vi "ini_object_save.vi"(7 "generate error if unsuppoted data type (true)":bool=TRUE, 8 "error in":errorcluster, 10 "auto ini row":T1, 11 "refnum in":T2) -> (0 "error out":errorcluster, 3 "refnum out":T2)   [LabVIEW 2020]
uses:
  <vilib>/Utility/config.llb/Config Data RefNum.ctl
  ini_parse_row.ctl
  <vilib>/Utility/config.llb/Write Key (String).vi
  <vilib>/Utility/config.llb/Write Key (Path).vi
  <vilib>/Utility/config.llb/Write Key (Boolean).vi
  <vilib>/Utility/config.llb/Write Key (I32).vi
  <vilib>/Utility/config.llb/Write Key (Double).vi
  <vilib>/Utility/config.llb/Write Key (U32).vi
  <vilib>/Utility/config.llb/NI_LVConfig.lvlib
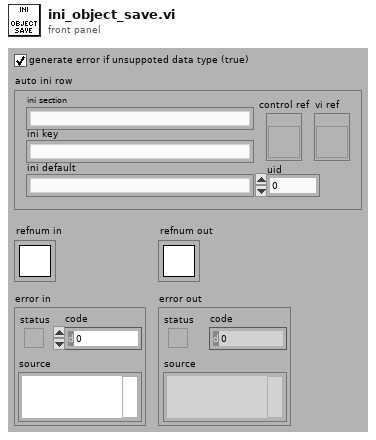
[diagram p1: front panel]
types:
  T1 = typedef "ini_parse_row.ctl" = cluster{"ini section":string, "ini key":string, "ini default":string, "control ref":refnum<vi>, "uid":i32, "vi ref":refnum<vi>}
  T2 = typedef "NI_LVConfig.lvlib/Config Data RefNum.ctl" = refnum<k1>
  T3 = cluster{"Value":string[][], "Row Headers[]":string[], "Column Headers[]":string[]}
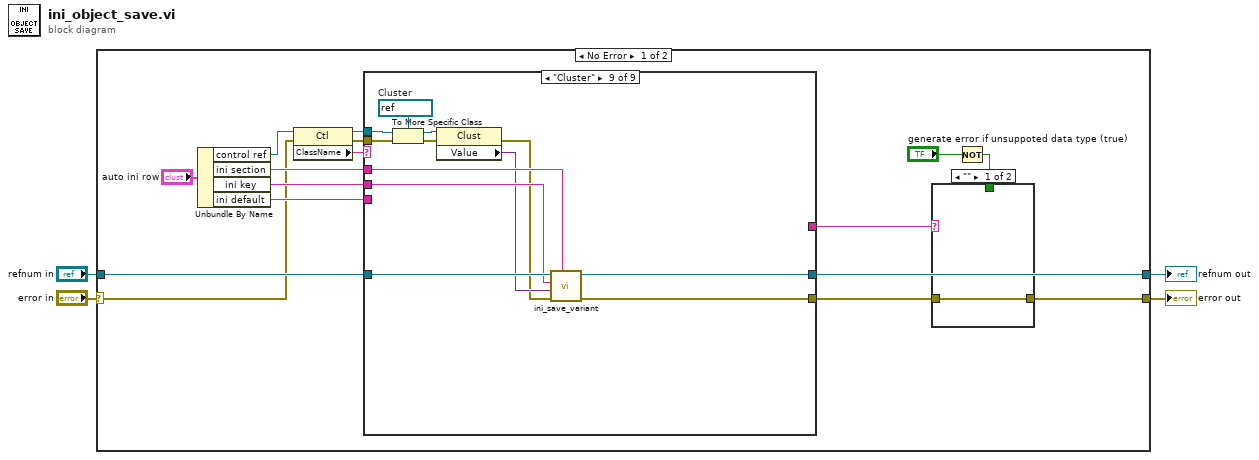
[diagram p0: block diagram]
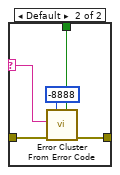
[diagram p2: hidden frame]
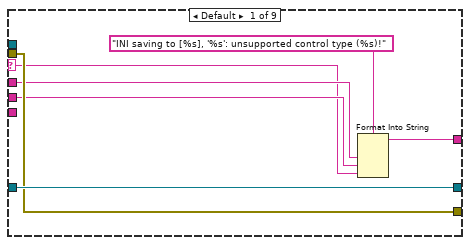
[diagram p3: hidden frame]
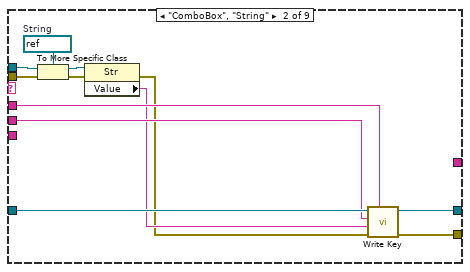
[diagram p4: hidden frame]
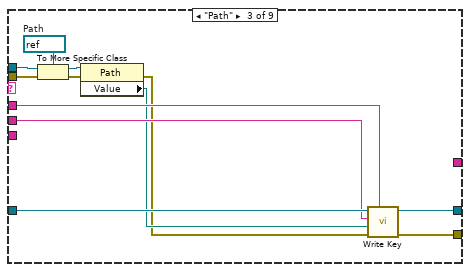
[diagram p5: hidden frame]
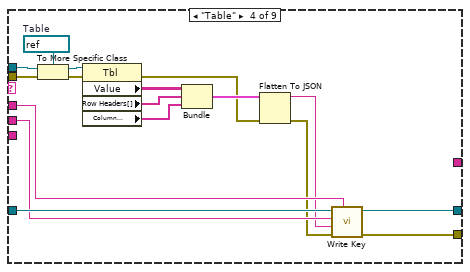
[diagram p6: hidden frame]
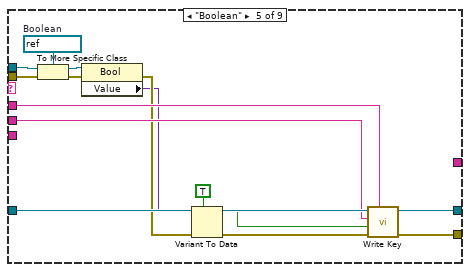
[diagram p7: hidden frame]
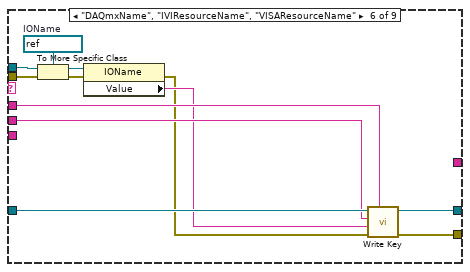
[diagram p8: hidden frame]
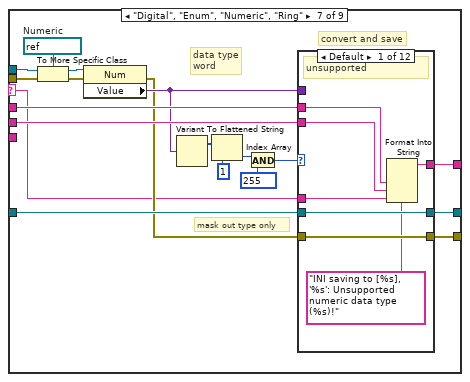
[diagram p9: hidden frame]
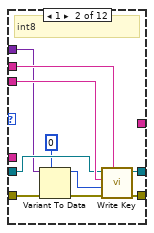
[diagram p10: hidden frame]
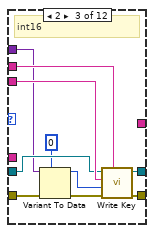
[diagram p11: hidden frame]
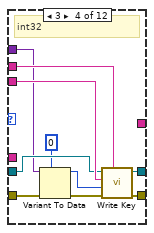
[diagram p12: hidden frame]
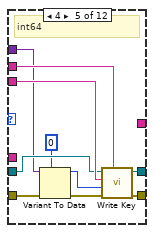
[diagram p13: hidden frame]
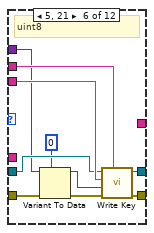
[diagram p14: hidden frame]
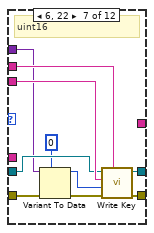
[diagram p15: hidden frame]
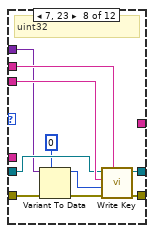
[diagram p16: hidden frame]
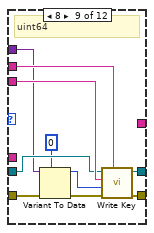
[diagram p17: hidden frame]
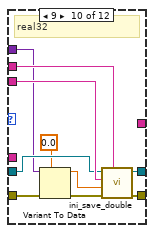
[diagram p18: hidden frame]
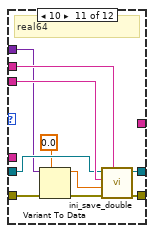
[diagram p19: hidden frame]
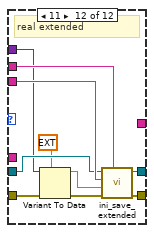
[diagram p20: hidden frame]
diagram:
  n1 = case shown="No Error" "error in" {
    selector: "error in" -> [w5 w424]
    tunnel: "refnum in" -> [w20 w423]
    tunnel: [w19 w423] -> w3
    tunnel: [w9 w424] -> w2
    frame No Error {
      n2 = Unbundle By Name("auto ini row") -> ("control ref"=w15:refnum<vi>, "ini section"=w17:string, "ini key"=w16:string, "ini default"=w13:string)
      n3 = property class="Ctl"(reference=w15, error in=w5) -> (reference out=w11:refnum<vi>, error out=w12:errorcluster, "ClassName"=w14:string)
      n4 = case shown="\"Cluster\"" w14 {
        selector: w14 -> [w27 _ _ _ _ _ w102 w243 _]
        tunnel: [w32 w45 w57 w74 w89 w101 w120 w253 w422] -> w10
        tunnel: w20 -> [w33 w44 w56 w73 w88 w100 w119 w252 w421]
        tunnel: [w33 w43 w55 w72 w87 w99 w118 w251 w420] -> w19
        tunnel: w17 -> [w29 w42 w54 w71 w86 w98 w117 w250 w419]
        tunnel: w16 -> [w28 w41 w53 w70 w85 w97 w116 w249 w418]
        tunnel: w13 -> [_ _ _ _ _ _ _ _ _]
        tunnel: w12 -> [w32 w38 w50 w67 w82 w94 w114 w247 w416]
        tunnel: w11 -> [_ w40 w52 w69 w84 w96 w115 w248 w417]
        tunnel: [w30 _ _ _ _ _ w103 _ _] -> w8
        frame Default {
          n5 = Format Into String(format string="INI saving to [%s], '%s': unsupported control type (%s)!", w29, w28, w27) -> (resulting string=w30:string)  [unwired: 2 in, 1 out]
        }
        frame "ComboBox", "String" {
          w36 = refnum<vi> refnum  # String
          n6 = To More Specific Class(target class=w36, reference=w40, error in=w38) -> (specific class reference=w39:refnum<vi>, error out=w37:errorcluster)
          n7 = property class="Str"(reference=w39, error in=w37) -> (error out=w34:errorcluster, "Value"=w35:string)  [unwired: 1 out]
          n8 = call-poly <vilib>:"Write Key.vi"("section"=w42, "error in (no error)"=w34, "value"=w35, "key"=w41, "refnum"=w44) -> ("error out"=w45:errorcluster, "refnum out"=w43:T2)  [unwired: 4 in, 1 out]
        }
        frame "Path" {
          w48 = refnum<vi> refnum  # Path
          n9 = To More Specific Class(target class=w48, reference=w52, error in=w50) -> (specific class reference=w51:refnum<vi>, error out=w49:errorcluster)
          n10 = property class="Path"(reference=w51, error in=w49) -> (error out=w46:errorcluster, "Value"=w47:path)  [unwired: 1 out]
          n11 = call-poly <vilib>:"Write Key.vi"("section"=w54, "error in (no error)"=w46, "value"=w47, "key"=w53, "refnum"=w56) -> ("error out"=w57:errorcluster, "refnum out"=w55:T2)  [unwired: 4 in, 1 out]
        }
        frame "Table" {
          w65 = refnum<vi> refnum  # Table
          n12 = To More Specific Class(target class=w65, reference=w69, error in=w67) -> (specific class reference=w68:refnum<vi>, error out=w66:errorcluster)
          n13 = property class="Tbl"(reference=w68, error in=w66) -> (error out=w60:errorcluster, "Value"=w64:string[][], "Row Headers[]"=w63:string[], "Column Headers[]"=w62:string[])  [unwired: 1 out]
          n14 = Bundle("Value"=w64, "Row Headers[]"=w63, "Column Headers[]"=w62) -> (w61:T3)  [unwired: 1 in]
          n15 = Flatten To JSON(anything=w61, error in (no error)=w60) -> (JSON string=w58:string, 11:w59:errorcluster)  [unwired: 1 in]
          n16 = call-poly <vilib>:"Write Key.vi"("section"=w71, "error in (no error)"=w59, "value"=w58, "key"=w70, "refnum"=w73) -> ("error out"=w74:errorcluster, "refnum out"=w72:T2)  [unwired: 4 in, 1 out]
        }
        frame "Boolean" {
          w80 = refnum<vi> refnum  # Boolean
          n17 = To More Specific Class(target class=w80, reference=w84, error in=w82) -> (specific class reference=w83:refnum<vi>, error out=w81:errorcluster)
          n18 = property class="Bool"(reference=w83, error in=w81) -> (error out=w79:errorcluster, "Value"=w76:variant)  [unwired: 1 out]
          n19 = Variant To Data(error in=w79, type=TRUE, Variant=w76) -> (data=w77:bool, error out=w78:errorcluster)
          n20 = call-poly <vilib>:"Write Key.vi"("section"=w86, "error in (no error)"=w78, "value"=w77, "key"=w85, "refnum"=w88) -> ("error out"=w89:errorcluster, "refnum out"=w87:T2)  [unwired: 4 in, 1 out]
        }
        frame "DAQmxName", "IVIResourceName", "VISAResourceName" {
          w92 = refnum<vi> refnum  # IOName
          n21 = To More Specific Class(target class=w92, reference=w96, error in=w94) -> (specific class reference=w95:refnum<vi>, error out=w93:errorcluster)
          n22 = property class="IOName"(reference=w95, error in=w93) -> (error out=w90:errorcluster, "Value"=w91:string)  [unwired: 1 out]
          n23 = call-poly <vilib>:"Write Key.vi"("section"=w98, "error in (no error)"=w90, "value"=w91, "key"=w97, "refnum"=w100) -> ("error out"=w101:errorcluster, "refnum out"=w99:T2)  [unwired: 4 in, 1 out]
        }
        frame "Digital", "Enum", "Numeric", "Ring" {
          w113 = refnum<vi> refnum  # Numeric
          # "convert and save"
          # "data type\nword"
          # "mask out type only"
          n24 = To More Specific Class(target class=w113, reference=w115, error in=w114) -> (specific class reference=w111:refnum<vi>, error out=w112:errorcluster)
          n25 = property class="Num"(reference=w111, error in=w112) -> (error out=w104:errorcluster, "Value"=w105:variant)  [unwired: 1 out]
          n26 = Variant To Flattened String(Variant=w105) -> (1:w110:i16[])  [unwired: 1 out]
          n27 = Index Array(array=w110, index=1) -> (element=w108:i16)
          n28 = And(x=w108, y=i16 255) -> (x .and. y?=w107:i16)
          n29 = case shown="Default" w107 {
            tunnel: w104 -> [w126 w133 w143 w153 w163 w173 w183 w193 w203 w213 w223 w233]
            tunnel: [w126 w137 w147 w157 w167 w177 w187 w197 w207 w217 w227 w237] -> w120
            tunnel: w119 -> [w127 w130 w140 w150 w160 w170 w180 w190 w200 w211 w220 w230]
            tunnel: [w127 w136 w146 w156 w166 w176 w186 w196 w206 w216 w226 w236] -> w118
            tunnel: w117 -> [w123 w135 w145 w155 w165 w175 w185 w195 w205 w215 w225 w235]
            tunnel: w116 -> [w122 w134 w144 w154 w164 w174 w184 w194 w204 w214 w224 w234]
            tunnel: w105 -> [_ w129 w139 w149 w159 w169 w179 w189 w199 w210 w219 w229]
            tunnel: [w125 _ _ _ _ _ _ _ _ _ _ _] -> w103
            tunnel: w102 -> [w121 _ _ _ _ _ _ _ _ _ _ _]
            frame Default {
              # "unsupported"
              n30 = Format Into String(format string="INI saving to [%s], '%s': Unsupported numeric data type (%s)!", w123, w122, w121) -> (resulting string=w125:string)  [unwired: 2 in, 1 out]
            }
            frame 1 {
              # "int8"
              n31 = Variant To Data(error in=w133, type=i8 0, Variant=w129) -> (data=w131:i8, error out=w132:errorcluster)
              n32 = call-poly <vilib>:"Write Key.vi"("section"=w135, "error in (no error)"=w132, "value"=w131, "key"=w134, "refnum"=w130) -> ("error out"=w137:errorcluster, "refnum out"=w136:T2)  [unwired: 4 in, 1 out]
            }
            frame 2 {
              # "int16"
              n33 = Variant To Data(error in=w143, type=i16 0, Variant=w139) -> (data=w141:i16, error out=w142:errorcluster)
              n34 = call-poly <vilib>:"Write Key.vi"("section"=w145, "error in (no error)"=w142, "value"=w141, "key"=w144, "refnum"=w140) -> ("error out"=w147:errorcluster, "refnum out"=w146:T2)  [unwired: 4 in, 1 out]
            }
            frame 3 {
              # "int32"
              n35 = Variant To Data(error in=w153, type=0, Variant=w149) -> (data=w151:i32, error out=w152:errorcluster)
              n36 = call-poly <vilib>:"Write Key.vi"("section"=w155, "error in (no error)"=w152, "value"=w151, "key"=w154, "refnum"=w150) -> ("error out"=w157:errorcluster, "refnum out"=w156:T2)  [unwired: 4 in, 1 out]
            }
            frame 4 {
              # "int64"
              n37 = Variant To Data(error in=w163, type=i64 0, Variant=w159) -> (data=w161:i64, error out=w162:errorcluster)
              n38 = call-poly <vilib>:"Write Key.vi"("section"=w165, "error in (no error)"=w162, "value"=w161, "key"=w164, "refnum"=w160) -> ("error out"=w167:errorcluster, "refnum out"=w166:T2)  [unwired: 4 in, 1 out]
            }
            frame 5, 21 {
              # "uint8"
              n39 = Variant To Data(error in=w173, type=u8 0, Variant=w169) -> (data=w171:u8, error out=w172:errorcluster)
              n40 = call-poly <vilib>:"Write Key.vi"("section"=w175, "error in (no error)"=w172, "value"=w171, "key"=w174, "refnum"=w170) -> ("error out"=w177:errorcluster, "refnum out"=w176:T2)  [unwired: 4 in, 1 out]
            }
            frame 6, 22 {
              # "uint16"
              n41 = Variant To Data(error in=w183, type=u16 0, Variant=w179) -> (data=w181:u16, error out=w182:errorcluster)
              n42 = call-poly <vilib>:"Write Key.vi"("section"=w185, "error in (no error)"=w182, "value"=w181, "key"=w184, "refnum"=w180) -> ("error out"=w187:errorcluster, "refnum out"=w186:T2)  [unwired: 4 in, 1 out]
            }
            frame 7, 23 {
              # "uint32"
              n43 = Variant To Data(error in=w193, type=u32 0, Variant=w189) -> (data=w191:u32, error out=w192:errorcluster)
              n44 = call-poly <vilib>:"Write Key.vi"("section"=w195, "error in (no error)"=w192, "value"=w191, "key"=w194, "refnum"=w190) -> ("error out"=w197:errorcluster, "refnum out"=w196:T2)  [unwired: 4 in, 1 out]
            }
            frame 8 {
              # "uint64"
              n45 = Variant To Data(error in=w203, type=u64 0, Variant=w199) -> (data=w201:u64, error out=w202:errorcluster)
              n46 = call-poly <vilib>:"Write Key.vi"("section"=w205, "error in (no error)"=w202, "value"=w201, "key"=w204, "refnum"=w200) -> ("error out"=w207:errorcluster, "refnum out"=w206:T2)  [unwired: 4 in, 1 out]
            }
            frame 9 {
              # "real32"
              n47 = Variant To Data(error in=w213, type=sgl 0.0, Variant=w210) -> (data=w208:sgl, error out=w212:errorcluster)
              n48 = call "ini_save_double.vi"("section"=w215, "error in"=w212, "double"=w208, "key"=w214, "refnum in"=w211) -> ("error out"=w217:errorcluster, "refnum out"=w216:T2)  [unwired: 4 in, 1 out]
            }
            frame 10 {
              # "real64"
              n49 = Variant To Data(error in=w223, type=0.0, Variant=w219) -> (data=w221:dbl, error out=w222:errorcluster)
              n50 = call "ini_save_double.vi"("section"=w225, "error in"=w222, "double"=w221, "key"=w224, "refnum in"=w220) -> ("error out"=w227:errorcluster, "refnum out"=w226:T2)  [unwired: 4 in, 1 out]
            }
            frame 11 {
              # "real extended"
              n51 = Variant To Data(error in=w233, type=ext 0.0, Variant=w229) -> (data=w231:ext, error out=w232:errorcluster)
              n52 = call "ini_save_extended.vi"("section"=w235, "error in"=w232, "double"=w231, "key"=w234, "refnum in"=w230) -> ("error out"=w237:errorcluster, "refnum out"=w236:T2)  [unwired: 4 in, 1 out]
            }
          }
        }
        frame "Array" {
          w246 = refnum<vi> refnum  # Array
          # "convert and save"
          n53 = To More Specific Class(target class=w246, reference=w248, error in=w247) -> (specific class reference=w244:refnum<vi>, error out=w245:errorcluster)
          n54 = property class="Arr"(reference=w244, error in=w245) -> (error out=w240:errorcluster, "Value"=w242:variant)  [unwired: 1 out]
          n55 = call "ini_object_parse_array.vi"("error in"=w240, "variant in"=w242) -> ("error out"=w239:errorcluster, "dims"=w238:i16, "type id"=w241:i16)  [unwired: 6 in, 1 out]
          n56 = case shown="1" w241 {
            tunnel: w239 -> [w263 w273 w283 w293 w299 w309 w319 w329 w339 w349 w359 w369 w379 w389 w399 w410]
            tunnel: [w260 w270 w280 w290 w303 w313 w323 w333 w343 w353 w363 w373 w383 w393 w403 w409] -> w253
            tunnel: w252 -> [w256 w266 w276 w286 w297 w307 w316 w326 w336 w346 w356 w366 w376 w386 w397 w407]
            tunnel: [w259 w269 w279 w289 w302 w312 w322 w332 w342 w352 w362 w372 w382 w392 w402 w408] -> w251
            tunnel: w250 -> [w257 w267 w277 w287 w301 w311 w321 w331 w341 w351 w361 w371 w381 w391 w401 w406]
            tunnel: w249 -> [w255 w265 w275 w285 w300 w310 w320 w330 w340 w350 w360 w370 w380 w390 w400 w405]
            tunnel: w242 -> [w262 w272 w282 w292 w296 w306 w315 w325 w335 w345 w355 w365 w375 w385 w396 w404]
            tunnel: w243 -> [_ _ _ _ _ _ _ _ _ _ _ _ _ _ _ _]
            tunnel: w238 -> [_ _ _ _ _ _ _ _ _ _ _ _ _ _ _ _]
            frame 1 {
              # "int8"
              n57 = Variant To Data(error in=w263, type=i8[] [], Variant=w262) -> (data=w254:i8[], error out=w258:errorcluster)
              n58 = call "ini_save_int64_vector.vi"("section"=w257, "error in"=w258, "values"=w254, "key"=w255, "refnum in"=w256) -> ("error out"=w260:errorcluster, "refnum out"=w259:T2)  [unwired: 4 in, 1 out]
            }
            frame 2 {
              # "int16"
              n59 = Variant To Data(error in=w273, type=i16[] [], Variant=w272) -> (data=w264:i16[], error out=w268:errorcluster)
              n60 = call "ini_save_int64_vector.vi"("section"=w267, "error in"=w268, "values"=w264, "key"=w265, "refnum in"=w266) -> ("error out"=w270:errorcluster, "refnum out"=w269:T2)  [unwired: 4 in, 1 out]
            }
            frame 3 {
              # "int32"
              n61 = Variant To Data(error in=w283, type=i32[] [], Variant=w282) -> (data=w274:i32[], error out=w278:errorcluster)
              n62 = call "ini_save_int64_vector.vi"("section"=w277, "error in"=w278, "values"=w274, "key"=w275, "refnum in"=w276) -> ("error out"=w280:errorcluster, "refnum out"=w279:T2)  [unwired: 4 in, 1 out]
            }
            frame 4 {
              # "int64"
              n63 = Variant To Data(error in=w293, type=i64[] [], Variant=w292) -> (data=w284:i64[], error out=w288:errorcluster)
              n64 = call "ini_save_int64_vector.vi"("section"=w287, "error in"=w288, "values"=w284, "key"=w285, "refnum in"=w286) -> ("error out"=w290:errorcluster, "refnum out"=w289:T2)  [unwired: 4 in, 1 out]
            }
            frame 5, 21 {
              # "uint8"
              n65 = Variant To Data(error in=w299, type=u8[] [], Variant=w296) -> (data=w294:u8[], error out=w298:errorcluster)
              n66 = call "ini_save_uint64_vector.vi"("section"=w301, "error in"=w298, "values"=w294, "key"=w300, "refnum in"=w297) -> ("error out"=w303:errorcluster, "refnum out"=w302:T2)  [unwired: 4 in, 1 out]
            }
            frame 6, 22 {
              # "uint16"
              n67 = Variant To Data(error in=w309, type=u16[] [], Variant=w306) -> (data=w304:u16[], error out=w308:errorcluster)
              n68 = call "ini_save_uint64_vector.vi"("section"=w311, "error in"=w308, "values"=w304, "key"=w310, "refnum in"=w307) -> ("error out"=w313:errorcluster, "refnum out"=w312:T2)  [unwired: 4 in, 1 out]
            }
            frame 7, 23 {
              # "uint32"
              n69 = Variant To Data(error in=w319, type=u32[] [], Variant=w315) -> (data=w317:u32[], error out=w318:errorcluster)
              n70 = call "ini_save_uint64_vector.vi"("section"=w321, "error in"=w318, "values"=w317, "key"=w320, "refnum in"=w316) -> ("error out"=w323:errorcluster, "refnum out"=w322:T2)  [unwired: 4 in, 1 out]
            }
            frame 8 {
              # "uint64"
              n71 = Variant To Data(error in=w329, type=u64[] [], Variant=w325) -> (data=w327:u64[], error out=w328:errorcluster)
              n72 = call "ini_save_uint64_vector.vi"("section"=w331, "error in"=w328, "values"=w327, "key"=w330, "refnum in"=w326) -> ("error out"=w333:errorcluster, "refnum out"=w332:T2)  [unwired: 4 in, 1 out]
            }
            frame 9 {
              # "real32"
              n73 = Variant To Data(error in=w339, type=sgl[] [], Variant=w335) -> (data=w337:sgl[], error out=w338:errorcluster)
              n74 = call "ini_save_double_vector.vi"("section"=w341, "error in"=w338, "values"=w337, "key"=w340, "refnum in"=w336) -> ("error out"=w343:errorcluster, "refnum out"=w342:T2)  [unwired: 4 in, 1 out]
            }
            frame 10 {
              # "real64"
              n75 = Variant To Data(error in=w349, type=dbl[] [], Variant=w345) -> (data=w347:dbl[], error out=w348:errorcluster)
              n76 = call "ini_save_double_vector.vi"("section"=w351, "error in"=w348, "values"=w347, "key"=w350, "refnum in"=w346) -> ("error out"=w353:errorcluster, "refnum out"=w352:T2)  [unwired: 4 in, 1 out]
            }
            frame 11 {
              # "real extended"
              n77 = Variant To Data(error in=w359, type=ext[] [], Variant=w355) -> (data=w357:ext[], error out=w358:errorcluster)
              n78 = call "ini_save_extended_vector.vi"("section"=w361, "error in"=w358, "values"=w357, "key"=w360, "refnum in"=w356) -> ("error out"=w363:errorcluster, "refnum out"=w362:T2)  [unwired: 4 in, 1 out]
            }
            frame 12 {
              # "cplx single"
              n79 = Variant To Data(error in=w369, type=csg[] [], Variant=w365) -> (data=w367:csg[], error out=w368:errorcluster)
              n80 = call "ini_save_cplx_double_vector.vi"("section"=w371, "error in"=w368, "values"=w367, "key"=w370, "refnum in"=w366) -> ("error out"=w373:errorcluster, "refnum out"=w372:T2)  [unwired: 4 in, 1 out]
            }
            frame 13 {
              # "cplx double"
              n81 = Variant To Data(error in=w379, type=cdb[] [], Variant=w375) -> (data=w377:cdb[], error out=w378:errorcluster)
              n82 = call "ini_save_cplx_double_vector.vi"("section"=w381, "error in"=w378, "values"=w377, "key"=w380, "refnum in"=w376) -> ("error out"=w383:errorcluster, "refnum out"=w382:T2)  [unwired: 4 in, 1 out]
            }
            frame 14 {
              # "cplx extended"
              n83 = Variant To Data(error in=w389, type=cxt[] [], Variant=w385) -> (data=w387:cxt[], error out=w388:errorcluster)
              n84 = call "ini_save_cplx_extended_vector.vi"("section"=w391, "error in"=w388, "values"=w387, "key"=w390, "refnum in"=w386) -> ("error out"=w393:errorcluster, "refnum out"=w392:T2)  [unwired: 4 in, 1 out]
            }
            frame 48, 55 {
              # "string"
              n85 = Variant To Data(error in=w399, type=string[] [], Variant=w396) -> (data=w394:string[], error out=w398:errorcluster)
              n86 = call "ini_save_string_vector.vi"("section"=w401, "error in"=w398, "values"=w394, "key"=w400, "refnum in"=w397) -> ("error out"=w403:errorcluster, "refnum out"=w402:T2)  [unwired: 4 in, 1 out]
            }
            frame Default {
              # "unknown"
              n87 = call "ini_save_variant.vi"("section"=w406, "error in"=w410, "Variant"=w404, "key"=w405, "refnum in"=w407) -> ("error out"=w409:errorcluster, "refnum out"=w408:T2)  [unwired: 4 in, 1 out]
            }
          }
        }
        frame "Cluster" {
          w415 = refnum<vi> refnum  # Cluster
          n88 = To More Specific Class(target class=w415, reference=w417, error in=w416) -> (specific class reference=w413:refnum<vi>, error out=w414:errorcluster)
          n89 = property class="Clust"(reference=w413, error in=w414) -> (error out=w411:errorcluster, "Value"=w412:variant)  [unwired: 1 out]
          n90 = call "ini_save_variant.vi"("section"=w419, "error in"=w411, "Variant"=w412, "key"=w418, "refnum in"=w421) -> ("error out"=w422:errorcluster, "refnum out"=w420:T2)  [unwired: 4 in, 1 out]
        }
      }
      n91 = Not(x="generate error if unsuppoted data type (true)") -> (.not. x?=w6:bool)
      n92 = case shown="\"\"" w8 {
        selector: w8 -> [_ w23]
        tunnel: w10 -> [w21 w26]
        tunnel: [w21 w25] -> w9
        tunnel: w6 -> [_ w22]
        frame "" {
        }
        frame Default {
          n93 = call <vilib>:"Error Cluster From Error Code.vi"("is warning? (False)"=w22, "error in (no error)"=w26, "error message (\"\")"=w23, "error code (0)"=-8888) -> ("error out"=w25:errorcluster)  [unwired: 5 in]
        }
      }
    }
    frame Error {
    }
  }
  "error out" <- w2
  "refnum out" <- w3
